vi "Read Multiple Direct.vi"(0 "VISA resource name":refnum<visa-resource-name>, 1 "All Data Elements (False)":bool, 2 "Timeout (30000 milliseconds)":u32=30000, 11 "error in (no error)":errorcluster) -> (4 "VISA resource name out":refnum<visa-resource-name>, 6 "Measurement Data":dbl[](array[numeric]), 8 "Time Stamp":string[](array[string]), 10 "Channel":string[](array[string]), 14 "Reading Number":string[](array[string]), 15 "error out":errorcluster)   [LabVIEW 2013, in "Keithley 27XX.lvlib"]
doc: "This VI initiates a reading, waits until data is available, and returns that data. The data is output directly to the bus instead of storing the data in the instruments internal data buffer.\n\nNote:\n(1) Returning all data elements requires ASCII transfers.\n\n(2) Timestamp, Channel, and Reading Number arrays will be left empty if the All Data Elements control is set to False."
uses:
  <instrlib>/Keithley 27XX/Keithley 27XX.lvlib
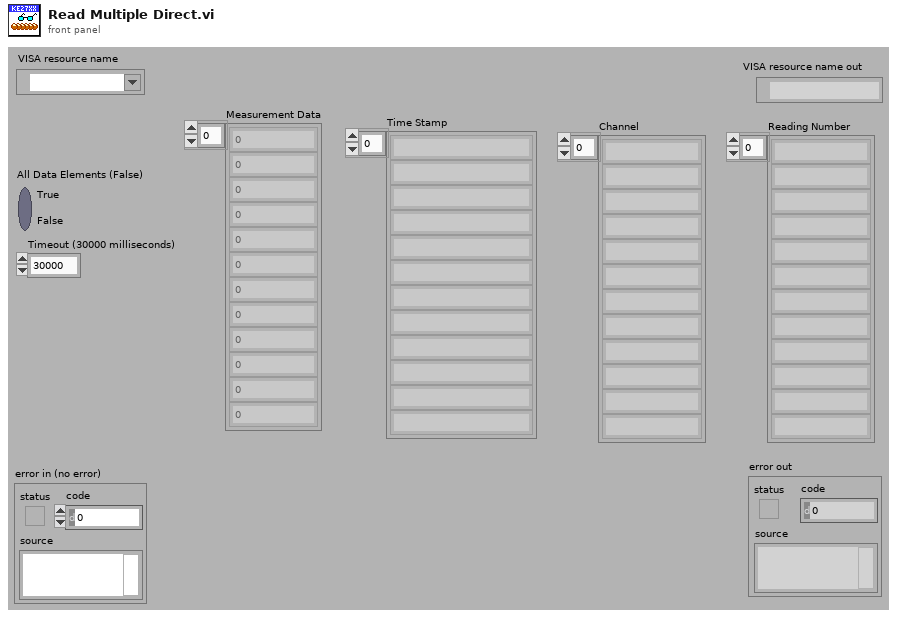
[diagram p1: front panel]
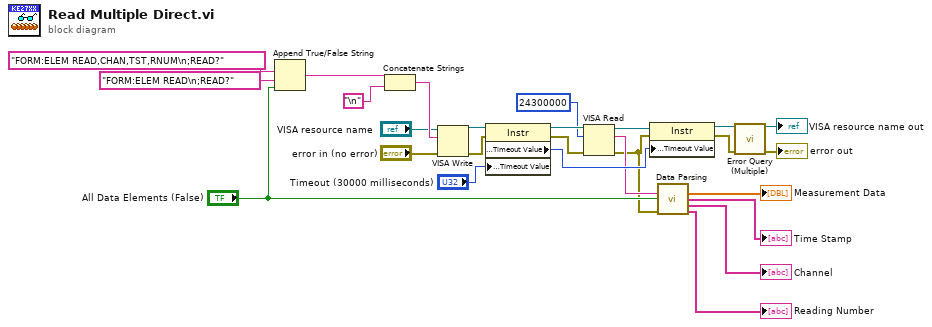
[diagram p0: block diagram]
diagram:
  n1 = Append True/False String(1:"All Data Elements (False)", 2:"FORM:ELEM READ\n;READ?", 3:"FORM:ELEM READ,CHAN,TST,RNUM\n;READ?" ("true string")) -> (0:w8:string)  [unwired: 1 in]
  n2 = Concatenate Strings(w8, "\n") -> (w24:string)
  n3 = VISA Write(VISA resource name="VISA resource name", write buffer=w24, error in (no error)="error in (no error)") -> (VISA resource name out=w15:refnum<visa-resource-name>, error out=w14:errorcluster)  [unwired: 1 out]
  n4 = property class="Instr"(reference=w15, error in=w14, "General Settings:Timeout Value"="Timeout (30000 milliseconds)") -> (reference out=w22:refnum<visa-resource-name>, error out=w21:errorcluster, "General Settings:Timeout Value"=w19:u32)
  n5 = VISA Read(VISA resource name=w22, byte count=u32 24300000, error in (no error)=w21) -> (VISA resource name out=w20:refnum<visa-resource-name>, read buffer=w3:string, error out=w1:errorcluster)  [unwired: 1 out]
  n6 = property class="Instr"(reference=w20, error in=w1, "General Settings:Timeout Value"=w19) -> (reference out=w12:refnum<visa-resource-name>, error out=w13:errorcluster)
  n7 = call <instrlib>:"Data Parsing.vi"("read buffer"=w3, "All Data Elements (False)"="All Data Elements (False)", "error in"=w1) -> ("Measurement Data"=→"Measurement Data":dbl[], "Time Stamp"=→"Time Stamp":string[], "Channel"=→"Channel":string[], "Reading Number"=→"Reading Number":string[])  [unwired: 9 in]
  n8 = call <instrlib>:"Error Query (Multiple).vi"("VISA resource name"=w12, "error in (no error)"=w13) -> ("VISA resource name out"=→"VISA resource name out":refnum<visa-resource-name>, "error out"=→"error out":errorcluster)  [unwired: 10 in, 2 out]
